vi "FGH Define.vi"(11 "Sampling Freqauency (Hz)":dbl=10000.0) -> (0 "G Matrix":T1, 1 "F  Matrix":T1=[[1.0, 0.0001], [0.0, 1.0]], 2 "Q = GQG'":T1, 3 "H Matrix":T1=[[0.0, 1.0], [9.81, 0.0]], 4 "R Matrix":T1=[[1e-10, 0.0], [0.0, 1e-11]])   [LabVIEW 2016]
uses:
  <vilib>/Analysis/Matrix/NI_Matrix.lvlib
  <vilib>/Analysis/Matrix/Numeric/Conversions/Array To Matrix - RA2.vi
  <vilib>/Analysis/Matrix/Datatypes/RealMatrix.ctl
  <vilib>/Analysis/NI_AALBase.lvlib
  <vilib>/Analysis/baseanly.llb/Real A x B.vi
  <vilib>/Analysis/NI_AALPro.lvlib
  <vilib>/Analysis/7linalg.llb/Real Transpose Matrix.vi
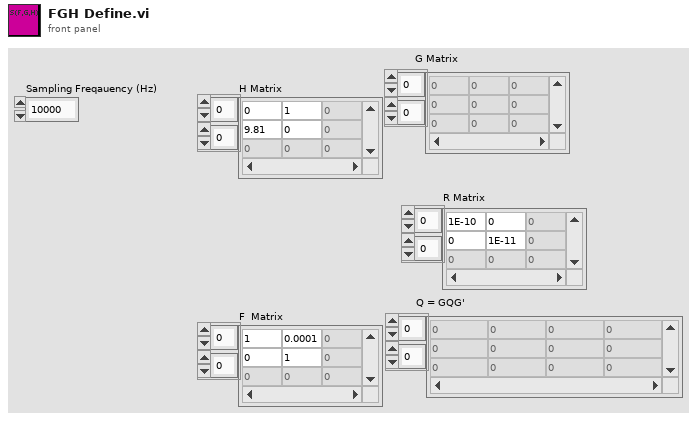
[diagram p1: front panel]
types:
  T1 = typedef "NI_Matrix.lvlib/RealMatrix.ctl" = dbl[][]
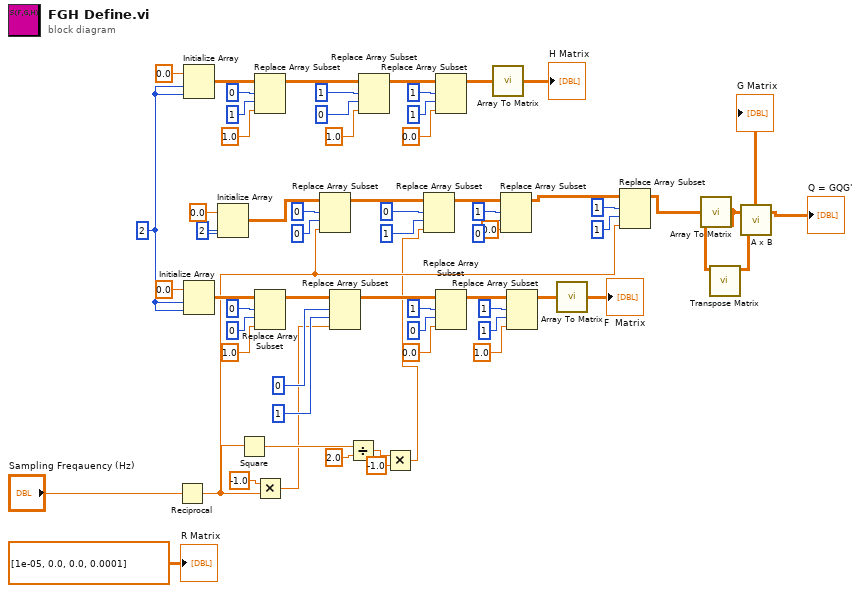
[diagram p0: block diagram]
diagram:
  w23 = 2 ("dimension size")
  w25 = 2 ("dimension size")
  n1 = Reciprocal(x="Sampling Freqauency (Hz)") -> (1/x=w8:dbl)
  n2 = Initialize Array(0.0 ("element"), w25, w25) -> (w51:dbl[][])
  n3 = Initialize Array(0.0 ("element"), w25, w25) -> (w30:dbl[][])
  n4 = Initialize Array(0.0 ("element"), w23, w23) -> (w14:dbl[][])
  n5 = Square(x=w8) -> (x^2=w45:dbl)
  n6 = Replace Array Subset(array=w51, new element=1.0 ("new element/subarray"), index (row)=0, index (col)=1 ("disabled index (col)")) -> (w55:dbl[][])
  n7 = Replace Array Subset(array=w30, new element=1.0 ("new element/subarray"), index (row)=0, index (col)=0 ("disabled index (col)")) -> (w34:dbl[][])
  n8 = Multiply(x=-1.0, y=w8) -> (x*y=w10:dbl)
  n9 = Replace Array Subset(array=w14, new element=w8, index (row)=0, index (col)=0 ("disabled index (col)")) -> (w18:dbl[][])
  n10 = Replace Array Subset(array=w34, new element=w10, index (row)=0, index (col)=1 ("disabled index (col)")) -> (w37:dbl[][])
  n11 = Divide(x=w45, y=2.0) -> (x/y=w6:dbl)
  n12 = Replace Array Subset(array=w55, new element=1.0 ("new element/subarray"), index (row)=1, index (col)=0 ("disabled index (col)")) -> (w59:dbl[][])
  n13 = Multiply(x=w6, y=-1.0) -> (x*y=w4:dbl)
  n14 = Replace Array Subset(array=w18, new element=w4, index (row)=0, index (col)=1 ("disabled index (col)")) -> (w15:dbl[][])
  n15 = Replace Array Subset(array=w59, new element=0.0 ("new element/subarray"), index (row)=1, index (col)=1 ("disabled index (col)")) -> (w62:dbl[][])
  n16 = Replace Array Subset(array=w37, new element=0.0 ("new element/subarray"), index (row)=1, index (col)=0 ("disabled index (col)")) -> (w41:dbl[][])
  n17 = call-poly <vilib>:"Array To Matrix.vi"("Real 2D Array"=w62) -> ("Real Matrix"=→"H Matrix":T1)
  n18 = Replace Array Subset(array=w15, new element=0.0 ("new element/subarray"), index (row)=1, index (col)=0 ("disabled index (col)")) -> (w11:dbl[][])
  n19 = Replace Array Subset(array=w41, new element=1.0 ("new element/subarray"), index (row)=1, index (col)=1 ("disabled index (col)")) -> (w60:dbl[][])
  n20 = call-poly <vilib>:"Array To Matrix.vi"("Real 2D Array"=w60) -> ("Real Matrix"=→"F  Matrix":T1)
  n21 = Replace Array Subset(array=w11, new element=w8, index (row)=1, index (col)=1 ("disabled index (col)")) -> (w7:dbl[][])
  n22 = call-poly <vilib>:"Array To Matrix.vi"("Real 2D Array"=w7) -> ("Real Matrix"=w2:T1)
  "G Matrix" <- w2
  n23 = call-poly <vilib>:"Transpose Matrix.vi"("Input Matrix"=w2) -> ("Matrix Transpose"=w1:T1)  [unwired: 9 in, 1 out]
  n24 = call-poly <vilib>:"A x B.vi"("B"=w1, "A"=w2) -> ("A x B"=→"Q = GQG'":T1)  [unwired: 1 out]
  "R Matrix" <- T1 [[1e-05, 0.0], [0.0, 0.0001]] ("F  Matrix")
